vi "Biometry Average2String Detail.vi"(8 "error in (no error)":errorcluster caption="错误输入（无错误）", 9 "Biometry Average Standard Deviation":T1, 10 "Biometry Average State":T2, 11 "Biometry Average Parameter":T3) -> (0 "error out":errorcluster caption="错误输出", 2 "Data Output":string[][](array[string]))   [LabVIEW 2015, in "Utility VIs.lvlib"]
doc: "该模板用于创建子VI。"
uses:
  Utility VIs.lvlib
  Database Processing/Support/Table/Biometry Average Parameter.ctl
  Database Processing/Support/Table/Biometry Average State.ctl
  Database Processing/Support/Table/Biometry Average Standard Deviation.ctl
  Database Processing/Database Processing.lvlib
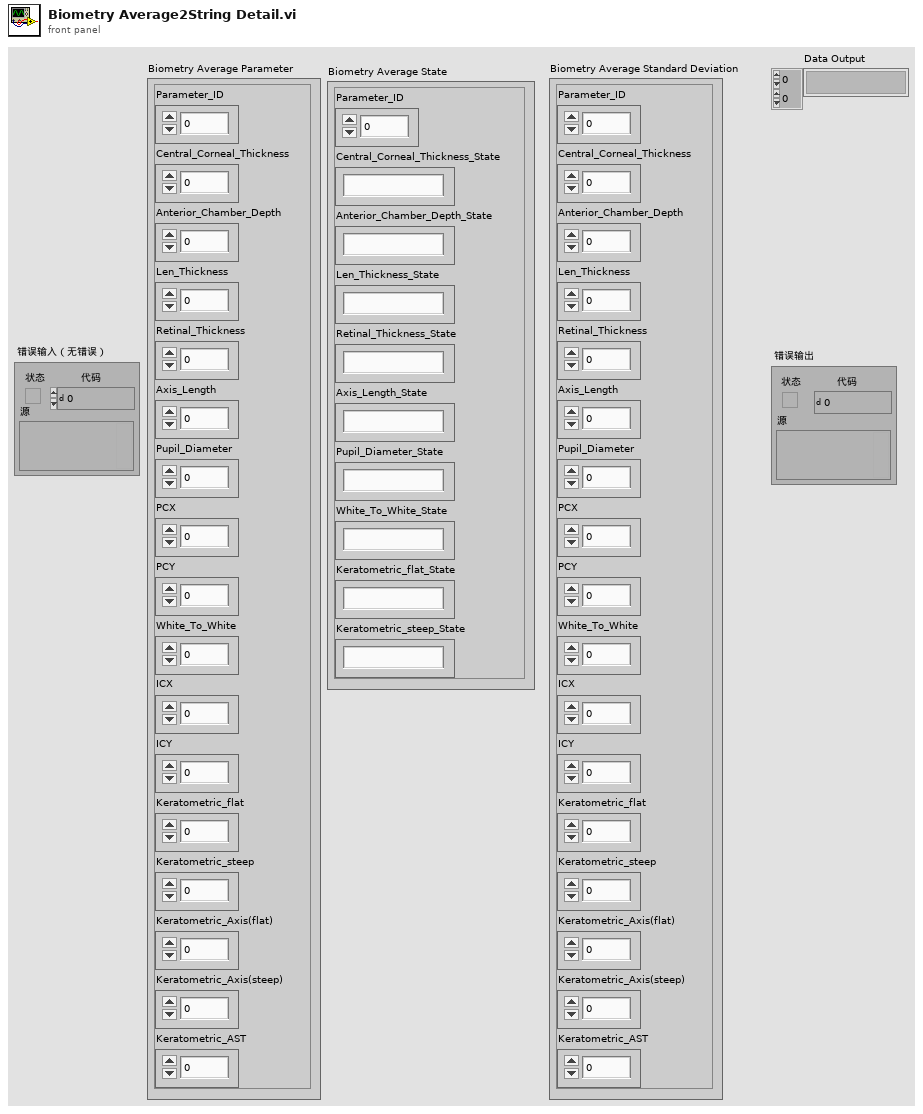
[diagram p1: front panel]
types:
  T1 = typedef "Database Processing.lvlib/Biometry Average Standard Deviation.ctl" = cluster{"Parameter_ID":i64, "Central_Corneal_Thickness":sgl, "Anterior_Chamber_Depth":sgl, "Len_Thickness":sgl, "Retinal_Thickness":sgl, "Axis_Length":sgl, "Pupil_Diameter":sgl, "PCX":sgl, "PCY":sgl, "White_To_White":sgl, "ICX":sgl, "ICY":sgl, "Keratometric_flat":sgl, "Keratometric_steep":sgl, "Keratometric_Axis(flat)":sgl, "Keratometric_Axis(steep)":sgl, "Keratometric_AST":sgl}
  T2 = typedef "Database Processing.lvlib/Biometry Average State.ctl" = cluster{"Parameter_ID":i64, "Central_Corneal_Thickness_State":string, "Anterior_Chamber_Depth_State":string, "Len_Thickness_State":string, "Retinal_Thickness_State":string, "Axis_Length_State":string, "Pupil_Diameter_State":string, "White_To_White_State":string, "Keratometric_flat_State":string, "Keratometric_steep_State":string}
  T3 = typedef "Database Processing.lvlib/Biometry Average Parameter.ctl" = cluster{"Parameter_ID":i64, "Central_Corneal_Thickness":sgl, "Anterior_Chamber_Depth":sgl, "Len_Thickness":sgl, "Retinal_Thickness":sgl, "Axis_Length":sgl, "Pupil_Diameter":sgl, "PCX":sgl, "PCY":sgl, "White_To_White":sgl, "ICX":sgl, "ICY":sgl, "Keratometric_flat":sgl, "Keratometric_steep":sgl, "Keratometric_Axis(flat)":sgl, "Keratometric_Axis(steep)":sgl, "Keratometric_AST":sgl}
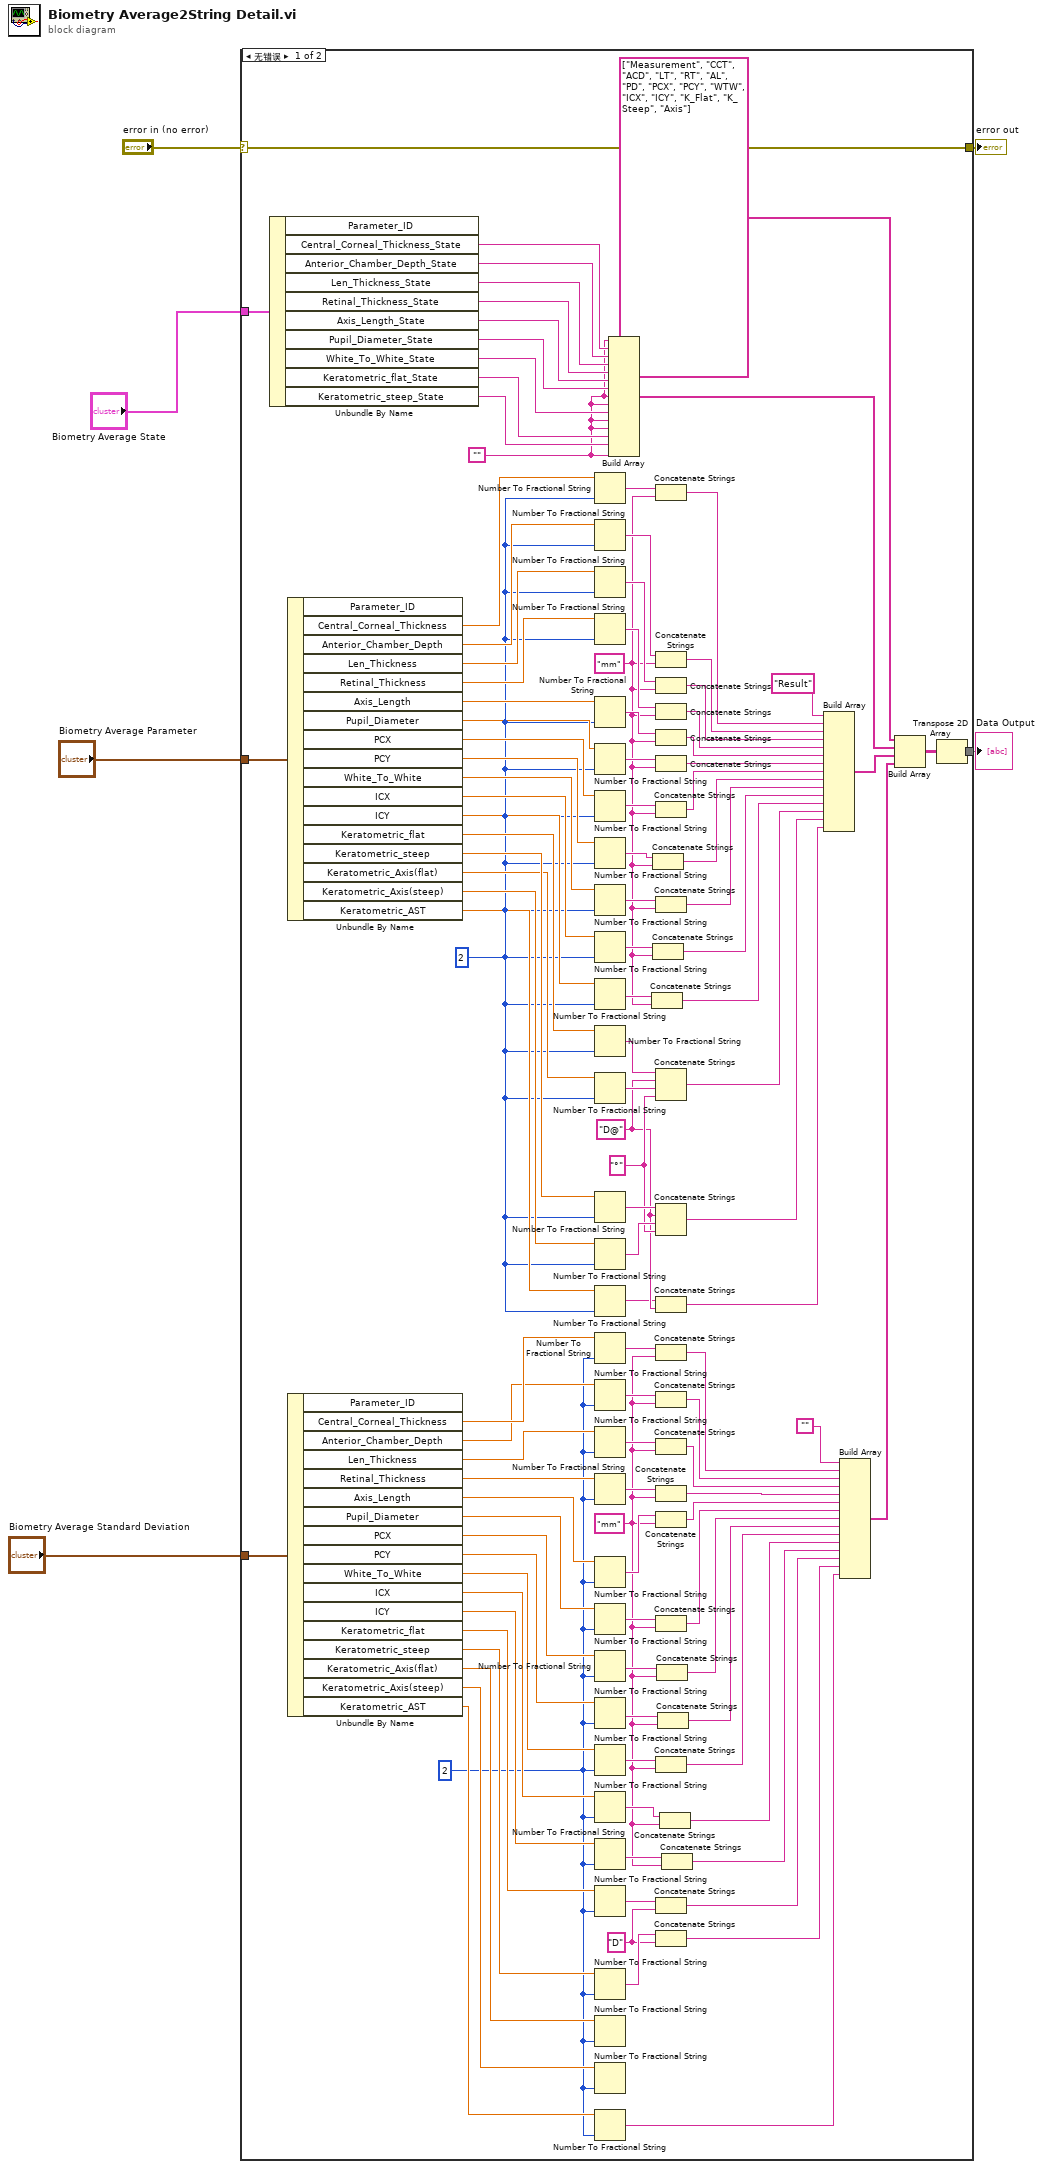
[diagram p0: block diagram]
diagram:
  n1 = case shown="无错误" "error in (no error)" {
    selector: "error in (no error)" -> [w44 w125]
    tunnel: [w44 w125] -> w5
    tunnel: "Biometry Average Parameter" -> [w124 _]
    tunnel: "Biometry Average Standard Deviation" -> [w123 _]
    tunnel: "Biometry Average State" -> [w122 _]
    tunnel: [w41 _] -> w1
    frame No Error {
      w9 = ""
      w66 = "D" ("字符串")
      w29 = "mm" ("字符串")
      w69 = i16 2 ("精度(6)")
      w79 = "°" ("字符串")
      w35 = "D@" ("字符串")
      w36 = "mm" ("字符串")
      w81 = i16 2 ("精度(6)")
      n2 = Unbundle By Name(w122) -> ("Central_Corneal_Thickness_State"=w65:string, "Anterior_Chamber_Depth_State"=w64:string, "Len_Thickness_State"=w63:string, "Retinal_Thickness_State"=w62:string, "Axis_Length_State"=w61:string, "Pupil_Diameter_State"=w60:string, "White_To_White_State"=w26:string, "Keratometric_flat_State"=w27:string, "Keratometric_steep_State"=w28:string)  [unwired: 1 out]
      n3 = Unbundle By Name(w124) -> ("Central_Corneal_Thickness"=w121:sgl, "Anterior_Chamber_Depth"=w120:sgl, "Len_Thickness"=w119:sgl, "Retinal_Thickness"=w118:sgl, "Axis_Length"=w117:sgl, "Pupil_Diameter"=w116:sgl, "PCX"=w115:sgl, "PCY"=w114:sgl, "White_To_White"=w113:sgl, "ICX"=w112:sgl, "ICY"=w111:sgl, "Keratometric_flat"=w110:sgl, "Keratometric_steep"=w109:sgl, "Keratometric_Axis(flat)"=w108:sgl, "Keratometric_Axis(steep)"=w83:sgl, "Keratometric_AST"=w82:sgl)  [unwired: 1 out]
      n4 = Unbundle By Name(w123) -> ("Central_Corneal_Thickness"=w107:sgl, "Anterior_Chamber_Depth"=w106:sgl, "Len_Thickness"=w105:sgl, "Retinal_Thickness"=w104:sgl, "Axis_Length"=w103:sgl, "Pupil_Diameter"=w102:sgl, "PCX"=w101:sgl, "PCY"=w100:sgl, "White_To_White"=w99:sgl, "ICX"=w98:sgl, "ICY"=w97:sgl, "Keratometric_flat"=w96:sgl, "Keratometric_steep"=w95:sgl, "Keratometric_Axis(flat)"=w94:sgl, "Keratometric_Axis(steep)"=w71:sgl, "Keratometric_AST"=w70:sgl)  [unwired: 1 out]
      n5 = Number To Fractional String(number=w121, precision (6)=w81) -> (F-format string=w93:string)  [unwired: 2 in]
      n6 = Number To Fractional String(number=w120, precision (6)=w81) -> (F-format string=w92:string)  [unwired: 2 in]
      n7 = Number To Fractional String(number=w119, precision (6)=w81) -> (F-format string=w91:string)  [unwired: 2 in]
      n8 = Number To Fractional String(number=w118, precision (6)=w81) -> (F-format string=w90:string)  [unwired: 2 in]
      n9 = Number To Fractional String(number=w117, precision (6)=w81) -> (F-format string=w89:string)  [unwired: 2 in]
      n10 = Number To Fractional String(number=w116, precision (6)=w81) -> (F-format string=w88:string)  [unwired: 2 in]
      n11 = Number To Fractional String(number=w115, precision (6)=w81) -> (F-format string=w40:string)  [unwired: 2 in]
      n12 = Number To Fractional String(number=w114, precision (6)=w81) -> (F-format string=w39:string)  [unwired: 2 in]
      n13 = Number To Fractional String(number=w113, precision (6)=w81) -> (F-format string=w87:string)  [unwired: 2 in]
      n14 = Number To Fractional String(number=w112, precision (6)=w81) -> (F-format string=w38:string)  [unwired: 2 in]
      n15 = Number To Fractional String(number=w111, precision (6)=w81) -> (F-format string=w37:string)  [unwired: 2 in]
      n16 = Number To Fractional String(number=w110, precision (6)=w81) -> (F-format string=w86:string)  [unwired: 2 in]
      n17 = Number To Fractional String(number=w108, precision (6)=w81) -> (F-format string=w84:string)  [unwired: 2 in]
      n18 = Number To Fractional String(number=w109, precision (6)=w81) -> (F-format string=w85:string)  [unwired: 2 in]
      n19 = Number To Fractional String(number=w83, precision (6)=w81) -> (F-format string=w80:string)  [unwired: 2 in]
      n20 = Number To Fractional String(number=w82, precision (6)=w81) -> (F-format string=w34:string)  [unwired: 2 in]
      n21 = Number To Fractional String(number=w107, precision (6)=w69) -> (F-format string=w78:string)  [unwired: 2 in]
      n22 = Number To Fractional String(number=w106, precision (6)=w69) -> (F-format string=w77:string)  [unwired: 2 in]
      n23 = Number To Fractional String(number=w105, precision (6)=w69) -> (F-format string=w76:string)  [unwired: 2 in]
      n24 = Number To Fractional String(number=w104, precision (6)=w69) -> (F-format string=w75:string)  [unwired: 2 in]
      n25 = Number To Fractional String(number=w103, precision (6)=w69) -> (F-format string=w74:string)  [unwired: 2 in]
      n26 = Number To Fractional String(number=w102, precision (6)=w69) -> (F-format string=w73:string)  [unwired: 2 in]
      n27 = Number To Fractional String(number=w101, precision (6)=w69) -> (F-format string=w33:string)  [unwired: 2 in]
      n28 = Number To Fractional String(number=w100, precision (6)=w69) -> (F-format string=w32:string)  [unwired: 2 in]
      n29 = Number To Fractional String(number=w99, precision (6)=w69) -> (F-format string=w72:string)  [unwired: 2 in]
      n30 = Number To Fractional String(number=w98, precision (6)=w69) -> (F-format string=w31:string)  [unwired: 2 in]
      n31 = Number To Fractional String(number=w97, precision (6)=w69) -> (F-format string=w30:string)  [unwired: 2 in]
      n32 = Number To Fractional String(number=w96, precision (6)=w69) -> (F-format string=w68:string)  [unwired: 2 in]
      n33 = Number To Fractional String(number=w95, precision (6)=w69) -> (F-format string=w67:string)  [unwired: 2 in]
      n34 = Number To Fractional String(number=w94, precision (6)=w69) -> ()  [unwired: 2 in, 1 out]
      n35 = Number To Fractional String(number=w71, precision (6)=w69) -> ()  [unwired: 2 in, 1 out]
      n36 = Number To Fractional String(number=w70, precision (6)=w69) -> (F-format string=w14:string)  [unwired: 2 in]
      n37 = Build Array(w9, w65, w64, w63, w62, w61, w60, w9, w9, w26, w9, w9, w27, w28, w9) -> (w47:string[])
      n38 = Concatenate Strings(w37, w36) -> (w21:string)
      n39 = Concatenate Strings(w39, w36) -> (w19:string)
      n40 = Concatenate Strings(w38, w36) -> (w20:string)
      n41 = Concatenate Strings(w93, w36) -> (w59:string)
      n42 = Concatenate Strings(w92, w36) -> (w58:string)
      n43 = Concatenate Strings(w91, w36) -> (w57:string)
      n44 = Concatenate Strings(w90, w36) -> (w56:string)
      n45 = Concatenate Strings(w89, w36) -> (w55:string)
      n46 = Concatenate Strings(w88, w36) -> (w54:string)
      n47 = Concatenate Strings(w40, w36) -> (w18:string)
      n48 = Concatenate Strings(w87, w36) -> (w23:string)
      n49 = Concatenate Strings(w86, w35, w84, w79) -> (w24:string)
      n50 = Concatenate Strings(w85, w35, w80, w79) -> (w25:string)
      n51 = Concatenate Strings(w34, w35) -> (w22:string)
      n52 = Concatenate Strings(w78, w29) -> (w53:string)
      n53 = Concatenate Strings(w77, w29) -> (w52:string)
      n54 = Concatenate Strings(w76, w29) -> (w51:string)
      n55 = Concatenate Strings(w75, w29) -> (w50:string)
      n56 = Concatenate Strings(w74, w29) -> (w49:string)
      n57 = Concatenate Strings(w73, w29) -> (w48:string)
      n58 = Concatenate Strings(w72, w29) -> (w15:string)
      n59 = Concatenate Strings(w68, w66) -> (w16:string)
      n60 = Concatenate Strings(w67, w66) -> (w17:string)
      n61 = Concatenate Strings(w33, w29) -> (w10:string)
      n62 = Concatenate Strings(w32, w29) -> (w11:string)
      n63 = Concatenate Strings(w31, w29) -> (w12:string)
      n64 = Concatenate Strings(w30, w29) -> (w13:string)
      n65 = Build Array("Result" ("元素"), w59, w58, w57, w56, w55, w54, w18, w19, w23, w20, w21, w24, w25, w22) -> (w45:string[])
      n66 = Build Array("", w53, w52, w51, w50, w49, w48, w10, w11, w15, w12, w13, w16, w17, w14) -> (w46:string[])
      n67 = Build Array(string[] ["Measurement", "CCT", "ACD", "LT", "RT", "AL", "PD", "PCX", "PCY", "WTW", "ICX", "ICY", "K_Flat", "K_Steep", "Axis"] ("元素"), w47, w45, w46) -> (w42:string[][])
      n68 = Transpose 2D Array(2D array=w42) -> (transposed array=w41:string[][])
    }
    frame Error {
    }
  }
  "error out" <- w5
  "Data Output" <- w1
